vi "Write to Execution Units.vi"(8 "error in (no error)":errorcluster, 11 "RT State Variables in":T1 {"Execution Unit Runtime Information"."Outgoing Data References"."Data Reference" format="%.0x"; "Execution Unit Runtime Information"."Incoming Data References" format="%.0x"}) -> (0 "error out":errorcluster, 3 "RT State Variables out":T1 {"Execution Unit Runtime Information"."Outgoing Data References"."Data Reference" format="%.0x"; "Execution Unit Runtime Information"."Incoming Data References" format="%.0x"})   [LabVIEW 2020, in "Communication Bus Template Engine.lvlib"]
uses:
  Communication Bus Template Engine.lvlib
  <vilib>/NI VeriStand/Custom Device API/Custom Device API.lvlib
  Includes/Communication Bus Interfaces.lvlibp/Execution Unit/Execution Unit/Execution Unit.lvclass
  <vilib>/NI/NIVS Inline Async API/_VS Inline Async API/VS Inline Async API/VS Inline Async API.lvclass
  RTStateVariables.ctl
  <vilib>/NI VeriStand/Custom Device API/Data Reference.ctl
  <vilib>/NI VeriStand/Custom Device API/Block Data Reference.ctl
  Execution Unit Runtime Information.ctl
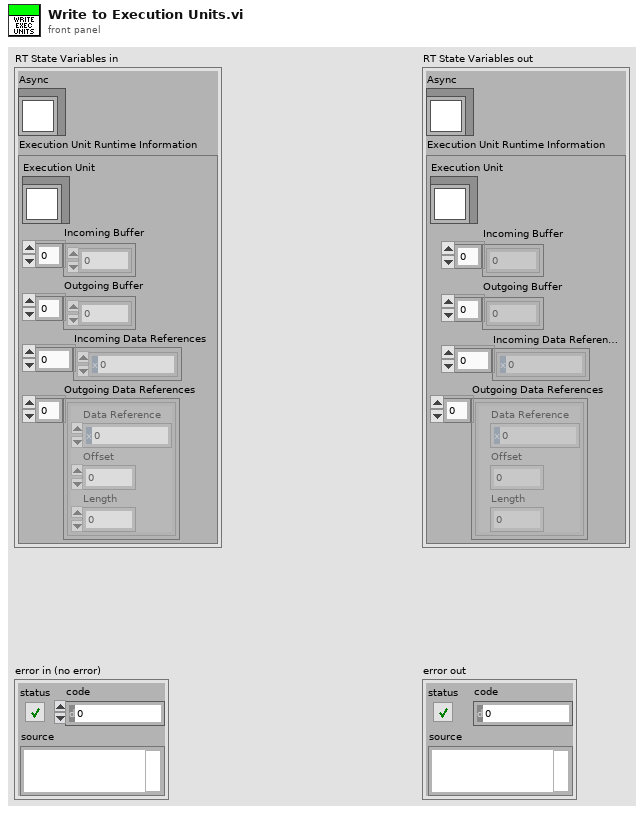
[diagram p1: front panel]
types:
  T1 = typedef "Communication Bus Template Engine.lvlib/RTStateVariables.ctl" = cluster{"Async":refnum<class "VS Inline Async API.lvclass">, "Execution Unit Runtime Information":T2}
  T2 = typedef "Communication Bus Template Engine.lvlib/Execution Unit Runtime Information.ctl" = cluster{"Execution Unit":refnum<class "Execution Unit.lvclass">, "Incoming Buffer":dbl[], "Outgoing Buffer":dbl[], "Incoming Data References":T3[], "Outgoing Data References":T4[]}
  T3 = typedef "Custom Device API.lvlib/Data Reference.ctl" = i32
  T4 = typedef "Custom Device API.lvlib/Block Data Reference.ctl" = cluster{"Data Reference":T3, "Offset":u64, "Length":u64}
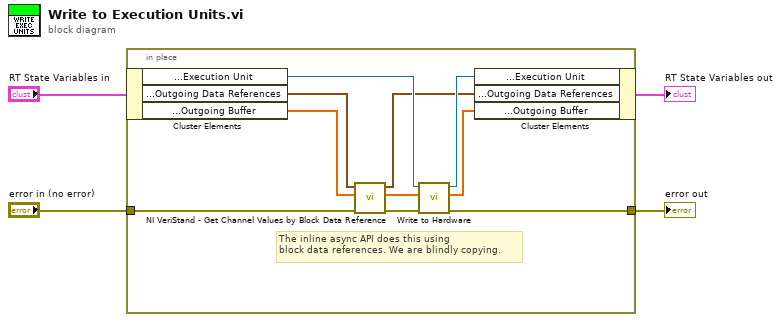
[diagram p0: block diagram]
diagram:
  n1 = in-place {
    in-place-border: "error in (no error)" -> [w10]
    in-place-border: [w11] -> w4
    # "The inline async API does this using\nblock data references. We are blindly copying."
    n2 = in-place-cluster #1("RT State Variables in") -> ("Execution Unit Runtime Information.Execution Unit"=w14:refnum<class "Execution Unit.lvclass">, "Execution Unit Runtime Information.Outgoing Data References"=w6:T4[], "Execution Unit Runtime Information.Outgoing Buffer"=w8:dbl[])
    n3 = call <vilib>:"NI VeriStand - Get Channel Values by Block Data Reference.vi"("error in (no error)"=w10, "Values Array in"=w8, "Block Data Ref"=w6) -> ("error out"=w9:errorcluster, "Values Array out"=w7:dbl[], "Block Data Ref dup"=w5:T4[])  [unwired: 6 in]
    n4 = call-dynamic "Write to Hardware.vi"("error in (no error)"=w9, "Values in"=w7, "Execution Unit in"=w14) -> ("error out"=w11:errorcluster, "Values out"=w12:dbl[], "Execution Unit out"=w13:refnum<class "Execution Unit.lvclass">)  [unwired: 6 in]
    n5 = in-place-cluster #1("Execution Unit Runtime Information.Execution Unit"=w13, "Execution Unit Runtime Information.Outgoing Data References"=w5, "Execution Unit Runtime Information.Outgoing Buffer"=w12) -> (→"RT State Variables out":T1)
  }
  "error out" <- w4
